vi "Show Databases.vi"(0 "InfluxDB in":refnum<class "Client.lvclass">, 11 "error in (no error)":errorcluster) -> (4 "InfluxDB out":refnum<class "Client.lvclass">, 6 "Database names":string[](array[string]), 15 "error out":errorcluster)   [LabVIEW 2018, in "InfluxDB Client.lvlib" / "Client.lvclass"]
doc: "Creates a database."
uses:
  Client.lvclass
  Results/Results.lvclass
  Results/Results.lvclass/Results.ctl
  Result/Result.lvclass/Result.ctl
  Series/Series.lvclass/Series.ctl
  <vilib>/LVH/i3 JSON/i3-json.lvlib
  Result/Result.lvclass
  Series/Series.lvclass
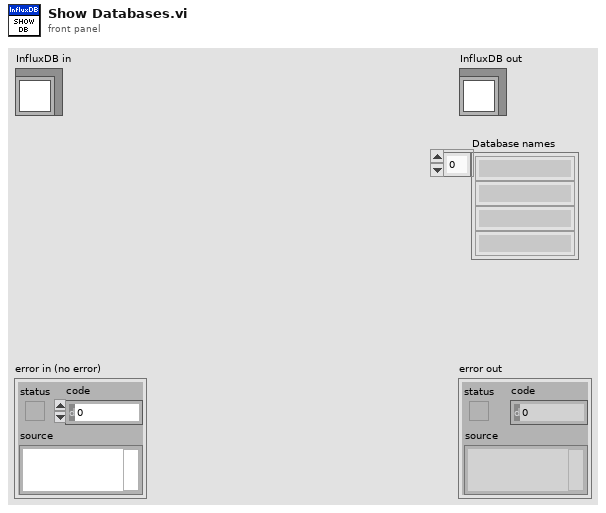
[diagram p1: front panel]
types:
  T1 = typedef "Dictionary Object RefNum__ogtk.ctl" = refnum<k1>
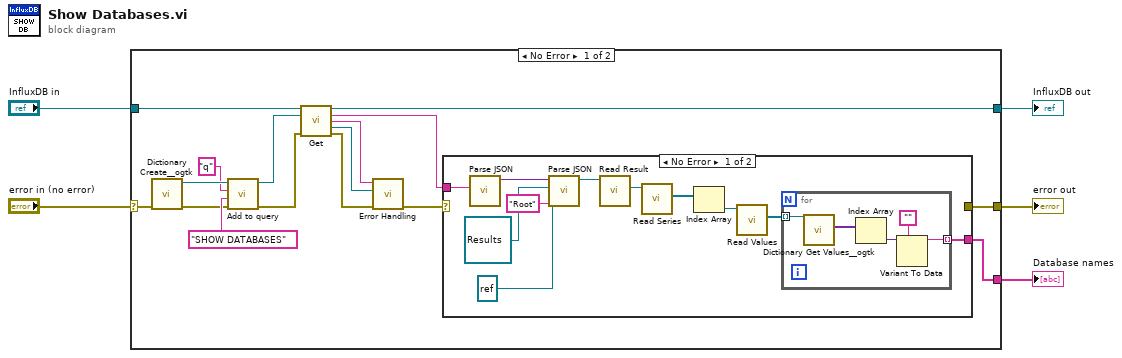
[diagram p0: block diagram]
diagram:
  n1 = case shown="No Error" "error in (no error)" {
    selector: "error in (no error)" -> [w15 w39]
    tunnel: [w20 w40] -> w3
    tunnel: "InfluxDB in" -> [w21 w40]
    tunnel: [w7 w39] -> w2
    tunnel: [w6 _] -> w1
    frame No Error {
      n2 = call <userlib>:"Dictionary Create__ogtk.vi"("error in (no error)"=w15) -> ("error out"=w13:errorcluster, "dictionary out"=w19:T1)  [unwired: 9 in]
      n3 = call "Add to query.vi"("error in (no error)"=w13, "Value"="SHOW DATABASES" ("Username"), "Parameter"="q" ("String"), "Query in"=w19) -> ("error out"=w16:errorcluster, "Query out"=w17:T1)  [unwired: 6 in]
      n4 = call "Get.vi"("InfluxDB Client in"=w21, "Query"=w17, "error in (no error)"=w16) -> ("InfluxDB Client out"=w20:refnum<class "Client.lvclass">, "body"=w12:string, "Status code"=w11:string, "Headers"=w9:T1, "error out"=w10:errorcluster)  [unwired: 8 in]
      n5 = call "Error Handling.vi"("error in (no error)"=w10, "HTTP headers"=w9, "HTTP status code"=w11) -> ("error out"=w8:errorcluster)  [unwired: 8 in]
      n6 = case shown="No Error" w8 {
        selector: w8 -> [_ w38]
        tunnel: w12 -> [w32 _]
        tunnel: [_ w38] -> w7
        tunnel: [w22 _] -> w6
        frame No Error {
          n7 = call <vilib>:"Parse JSON.vi"("JSON String"=w32) -> ("JSON Tree"=w31:variant)  [unwired: 7 in, 3 out]
          n8 = call <vilib>:"Parse JSON.vi"("Path"="Root", "Log File Ref"=refnum<file> refnum, "Results In"=refnum<class "Results.lvclass"> refnum, "JSON Tree"=w31) -> ("Results Out"=w23:refnum<class "Results.lvclass">)  [unwired: 7 in]
          n9 = call "Read Result.vi"("Results in"=w23) -> ("Result.lvclass"=w24:refnum<class "Result.lvclass">)  [unwired: 9 in, 1 out]
          n10 = call "Read Series.vi"("Result in"=w24) -> ("Series"=w25:refnum<class "Series.lvclass">[])  [unwired: 9 in, 1 out]
          n11 = Index Array(array=w25) -> (element=w26:refnum<class "Series.lvclass">)  [unwired: 1 in]
          n12 = call "Read Values.vi"("Series in"=w26) -> ("Values"=w27:T1[])  [unwired: 9 in, 1 out]
          n13 = for {
            tunnel: w27 -> [w37] mode=indexing
            tunnel: [w33] -> w22 mode=indexing
            n14 = call <userlib>:"Dictionary Get Values__ogtk.vi"("dictionary"=w37) -> ("values"=w36:variant[])  [unwired: 8 in, 2 out]
            n15 = Index Array(array=w36) -> (element=w35:variant)  [unwired: 1 in]
            n16 = Variant To Data(type="", Variant=w35) -> (data=w33:string)  [unwired: 1 in, 1 out]
          }
        }
        frame Error {
        }
      }
    }
    frame Error {
    }
  }
  "error out" <- w2
  "InfluxDB out" <- w3
  "Database names" <- w1
